vi "Vision VI - Knox.vi"(0 "Image In":T2, 7 "error in":errorcluster) -> (20 "Image Out":T2, 21 "Number of Particles (Particle Analysis 1)":i32, 24 "Particles":T1(array[cluster]), 27 "error out":errorcluster)   [LabVIEW 2014]
uses:
  <vilib>/vision/Image Controls.llb/IMAQ Image.ctl
  <vilib>/vision/NI_Vision_Development_Module.lvlib
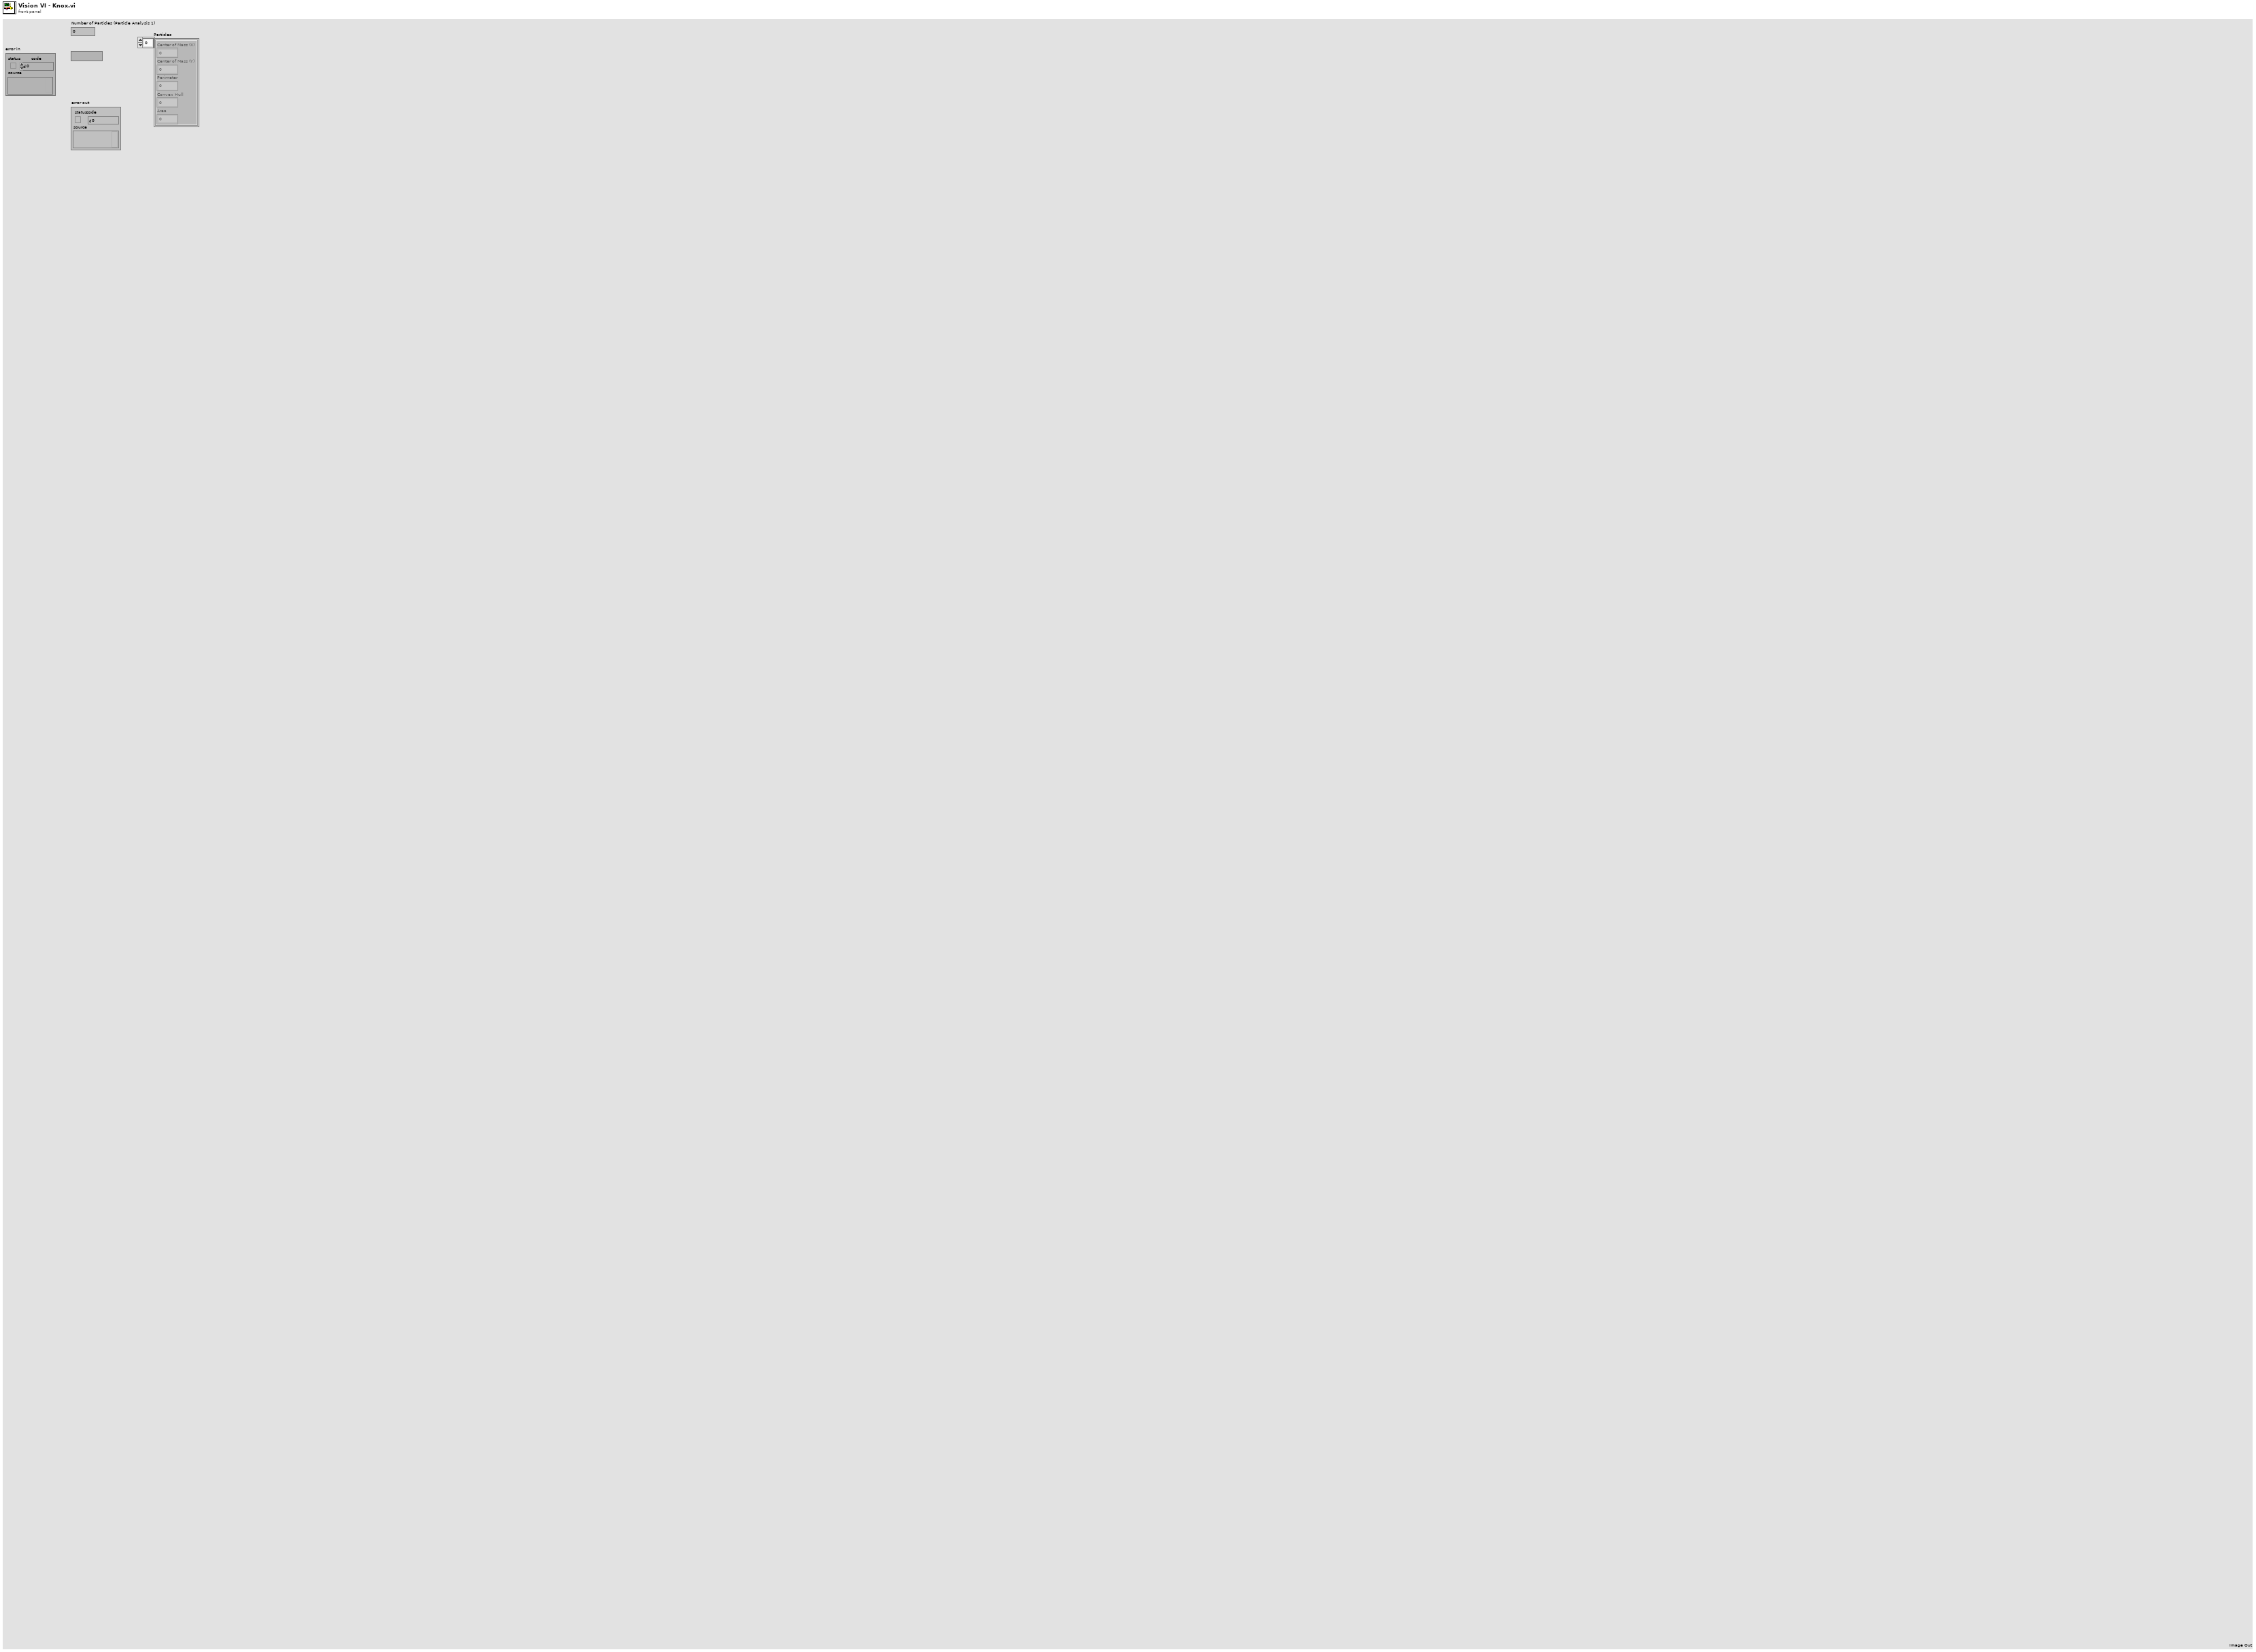
[diagram p1: front panel]
types:
  T1 = cluster{"Center of Mass (X)":dbl, "Center of Mass (Y)":dbl, "Perimeter":dbl, "Convex Hull":dbl, "Area":dbl}[]
  T2 = typedef "IMAQ Image.ctl" = refnum<image>
  T3 = cluster{"Center of Mass (X)":dbl, "Center of Mass (Y)":dbl, "Perimeter":dbl, "Convex Hull":dbl, "Area":dbl}
  T4 = enum32{"AutoM", "Close", "Dilate", "Erode", "Gradient", "Gradient out", "Gradient in", "Hit miss", "Open", "PClose", "POpen", "Thick", "Thin"}
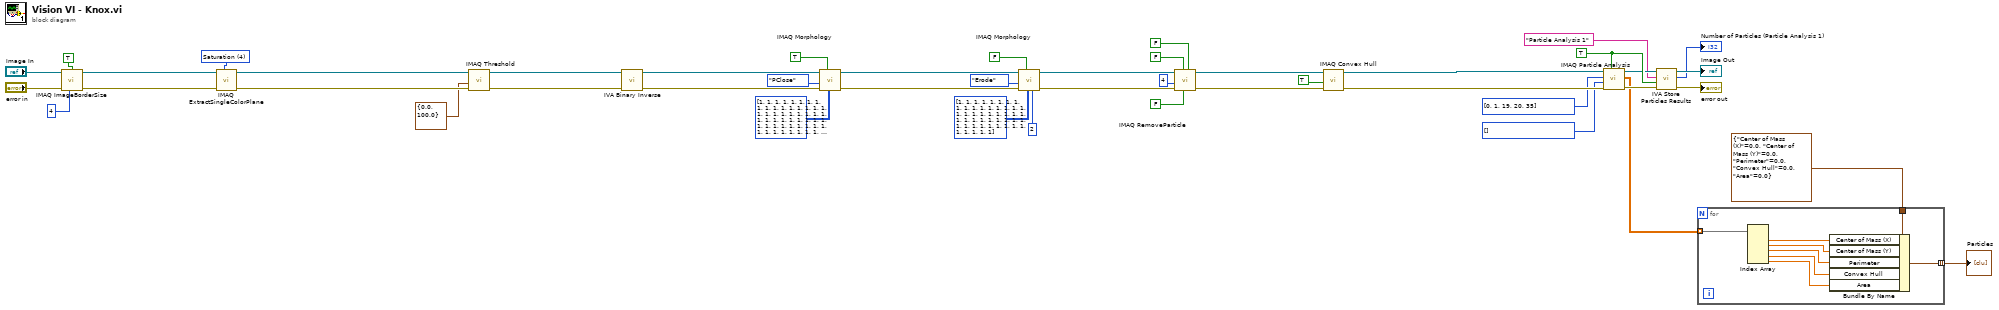
[diagram p0: block diagram]
diagram:
  w12 = i32[] [] items=["Center of Mass X", "Center of Mass Y", "First Pixel X", "First Pixel Y", "Bounding Rect Left", "Bounding Rect Top", "Bounding Rect Right", "Bounding Rect Bottom", "Max Feret Diameter Start X", "Max Feret Diameter Start Y", "Max Feret Diameter End X", "Max Feret Diameter End Y", "Max Horiz. Segment Length Left", "Max Horiz. Segment Length Right", "Max Horiz. Segment Length Row", "-", "Bounding Rect Width", "Bounding Rect Height", "Bounding Rect Diagonal", "Perimeter", "Convex Hull Perimeter", "Holes' Perimeter", "Max Feret Diameter", "Equivalent Ellipse Major Axis", "Equivalent Ellipse Minor Axis", "Equivalent Ellipse Minor Axis (Feret)", "Equivalent Rect Long Side", "Equivalent Rect Short Side", "Equivalent Rect Diagonal", "Equivalent Rect Short Side (Feret)", "Average Horiz. Segment Length", "Average Vert. Segment Length", "Hydraulic Radius", "Waddel Disk Diameter", "-", "Area", "Holes' Area", "Particle & Holes' Area", "Convex Hull Area", "Image Area", "-", "Number of Holes", "Number of Horiz. Segments", "Number of Vert. Segments", "-", "Orientation", "Max Feret Diameter Orientation", "-", "% Area/Image Area", "% Area/(Particle & Holes' Area)", "Ratio of Equivalent Ellipse Axes", "Ratio of Equivalent Rect Sides", "-", "Elongation Factor", "Compactness Factor", "Heywood Circularity Factor", "Type Factor", "-", "Sum X", "Sum Y", "Sum XX", "Sum XY", "Sum YY", "Sum XXX", "Sum XXY", "Sum XYY", "Sum YYY", "-", "Moment of Inertia XX", "Moment of Inertia XY", "Moment of Inertia YY", "Moment of Inertia XXX", "Moment of Inertia XXY", "Moment of Inertia XYY", "Moment of Inertia YYY", "Norm. Moment of Inertia XX", "Norm. Moment of Inertia XY", "Norm. Moment of Inertia YY", "Norm. Moment of Inertia XXX", "Norm. Moment of Inertia XXY", "Norm. Moment of Inertia XYY", "Norm. Moment of Inertia YYY", "Hu Moment 1", "Hu Moment 2", "Hu Moment 3", "Hu Moment 4", "Hu Moment 5", "Hu Moment 6", "Hu Moment 7"] ("Real-World Measurements")
  w13 = i32[] [0, 1, 19, 20, 35] items=["Center of Mass X", "Center of Mass Y", "First Pixel X", "First Pixel Y", "Bounding Rect Left", "Bounding Rect Top", "Bounding Rect Right", "Bounding Rect Bottom", "Max Feret Diameter Start X", "Max Feret Diameter Start Y", "Max Feret Diameter End X", "Max Feret Diameter End Y", "Max Horiz. Segment Length Left", "Max Horiz. Segment Length Right", "Max Horiz. Segment Length Row", "-", "Bounding Rect Width", "Bounding Rect Height", "Bounding Rect Diagonal", "Perimeter", "Convex Hull Perimeter", "Holes' Perimeter", "Max Feret Diameter", "Equivalent Ellipse Major Axis", "Equivalent Ellipse Minor Axis", "Equivalent Ellipse Minor Axis (Feret)", "Equivalent Rect Long Side", "Equivalent Rect Short Side", "Equivalent Rect Diagonal", "Equivalent Rect Short Side (Feret)", "Average Horiz. Segment Length", "Average Vert. Segment Length", "Hydraulic Radius", "Waddel Disk Diameter", "-", "Area", "Holes' Area", "Particle & Holes' Area", "Convex Hull Area", "Image Area", "-", "Number of Holes", "Number of Horiz. Segments", "Number of Vert. Segments", "-", "Orientation", "Max Feret Diameter Orientation", "-", "% Area/Image Area", "% Area/(Particle & Holes' Area)", "Ratio of Equivalent Ellipse Axes", "Ratio of Equivalent Rect Sides", "-", "Elongation Factor", "Compactness Factor", "Heywood Circularity Factor", "Type Factor", "-", "Sum X", "Sum Y", "Sum XX", "Sum XY", "Sum YY", "Sum XXX", "Sum XXY", "Sum XYY", "Sum YYY", "-", "Moment of Inertia XX", "Moment of Inertia XY", "Moment of Inertia YY", "Moment of Inertia XXX", "Moment of Inertia XXY", "Moment of Inertia XYY", "Moment of Inertia YYY", "Norm. Moment of Inertia XX", "Norm. Moment of Inertia XY", "Norm. Moment of Inertia YY", "Norm. Moment of Inertia XXX", "Norm. Moment of Inertia XXY", "Norm. Moment of Inertia XYY", "Norm. Moment of Inertia YYY", "Hu Moment 1", "Hu Moment 2", "Hu Moment 3", "Hu Moment 4", "Hu Moment 5", "Hu Moment 6", "Hu Moment 7"] ("Pixel Measurements")
  w10 = TRUE ("Connectivity 4/8 (8)")
  w41 = 4 items=["Red", "Green", "Blue", "Hue", "Saturation", "Luminance", "Value", "Intensity"] ("Color Plane")
  n1 = call "IMAQ ImageBorderSize"("Get/Set Status? (Set)"=TRUE, "Image"="Image In", "Image border size in"=4 ("Border Size"), "error in (no error)"="error in") -> ("Image Out"=w40:T2, "error out"=w44:errorcluster)  [unwired: 1 out]
  n2 = call "IMAQ ExtractSingleColorPlane"("Color Plane"=w41, "error in (no error)"=w44, "Image Src"=w40) -> ("error out"=w39:errorcluster, "Image Dst Out"=w37:T2)  [unwired: 1 in, 6 out]
  n3 = call "IMAQ Threshold"("error in (no error)"=w39, "Range"=cluster{"Lower value":sgl, "Upper value":sgl} {"Lower value"=0.0, "Upper value"=100.0}, "Image Src"=w37) -> ("error out"=w36:errorcluster, "Image Dst Out"=w35:T2)  [unwired: 3 in, 4 out]
  n4 = call <vilib>:"IVA Binary Inverse.vi"("error in (no error)"=w36, "Image In"=w35) -> ("error out"=w34:errorcluster, "Image Out"=w30:T2)  [unwired: 8 out]
  n5 = call "IMAQ Morphology"("Structuring Element"=i32[][] [[1, 1, 1, 1, 1, 1, 1, 1, 1], [1, 1, 1, 1, 1, 1, 1, 1, 1], [1, 1, 1, 1, 1, 1, 1, 1, 1], [1, 1, 1, 1, 1, 1, 1, 1, 1], [1, 1, 1, 1, 1, 1, 1, 1, 1], [1, 1, 1, 1, 1, 1, 1, 1, 1], [1, 1, 1, 1, 1, 1, 1, 1, 1], [1, 1, 1, 1, 1, 1, 1, 1, 1], [1, 1, 1, 1, 1, 1, 1, 1, 1]], "Square/Hexa (Square)"=TRUE, "error in (no error)"=w34, "Operation"=T4."PClose", "Image Src"=w30) -> ("error out"=w29:errorcluster, "Image Dst Out"=w24:T2)  [unwired: 2 in, 3 out]
  n6 = call "IMAQ Morphology"("Number of iterations (1)"=2, "Structuring Element"=i32[][] [[1, 1, 1, 1, 1, 1, 1], [1, 1, 1, 1, 1, 1, 1], [1, 1, 1, 1, 1, 1, 1], [1, 1, 1, 1, 1, 1, 1], [1, 1, 1, 1, 1, 1, 1], [1, 1, 1, 1, 1, 1, 1], [1, 1, 1, 1, 1, 1, 1]], "Square/Hexa (Square)"=FALSE, "error in (no error)"=w29, "Operation"=T4."Erode", "Image Src"=w24) -> ("error out"=w23:errorcluster, "Image Dst Out"=w18:T2)  [unwired: 1 in, 3 out]
  n7 = call "IMAQ RemoveParticle"("Connectivity 4/8 (8)"=FALSE, "Low Pass/High Pass (Low)"=FALSE, "Square/Hexa (Square)"=FALSE, "error in (no error)"=w23, "Number of Erosion"=4, "Image Src"=w18) -> ("error out"=w17:errorcluster, "Image Dst Out"=w16:T2)  [unwired: 1 in, 3 out]
  n8 = call "IMAQ Convex Hull"("error in (no error)"=w17, "Connectivity 4/8 (8)"=TRUE, "Image Src"=w16) -> ("error out"=w14:errorcluster, "Image Dst Out"=w11:T2)  [unwired: 1 in, 6 out]
  n9 = call "IMAQ Particle Analysis"("Connectivity 4/8 (8)"=w10, "error in (no error)"=w14, "Real-World Measurements"=w12, "Pixel Measurements"=w13, "Image"=w11) -> ("error out"=w6:errorcluster, "Particle Measurements (Pixels)"=w1:dbl[][], "Image Out (duplicate)"=w9:T2)  [unwired: 4 out]
  n10 = call <vilib>:"IVA Store Particles Results.vi"("error in (no error)"=w6, "Connectivity 4/8 (8)"=w10, "Step Name"="Particle Analysis 1", "Image in"=w9) -> ("error out"=→"error out":errorcluster, "Number of Particles"=→"Number of Particles (Particle Analysis 1)":i32, "Image dup"=→"Image Out":T2)  [unwired: 5 out]
  n11 = for {
    tunnel: w1 -> [w54] mode=indexing
    tunnel: T3 {"Center of Mass (X)"=0.0, "Center of Mass (Y)"=0.0, "Perimeter"=0.0, "Convex Hull"=0.0, "Area"=0.0} ("input cluster") -> [w53]
    tunnel: [w52] -> w2 mode=indexing
    n12 = Index Array(array=w54) -> (element #1=w51:dbl, element #2=w50:dbl, element #3=w49:dbl, element #4=w48:dbl, element #5=w47:dbl)  [unwired: 5 in]
    n13 = Bundle By Name(cluster=w53, "Center of Mass (X)"=w51, "Center of Mass (Y)"=w50, "Perimeter"=w49, "Convex Hull"=w48, "Area"=w47) -> (w52:T3)
  }
  "Particles" <- w2
